vi "Read String Direct.vi"(8 "error in (no error)":errorcluster, 9 "Timeout (ms)":i32, 11 "CIFTag in":refnum<class "CIF_CIPC_Chn_String.lvclass">) -> (0 "error out":errorcluster, 1 "timed out?":bool, 2 "Data":string, 3 "CIFTag out":refnum<class "CIF_CIPC_Chn_String.lvclass">)   [LabVIEW 2021, in "CIF_CIPC_Chn_String.lvclass"]
uses:
  CIF_CIPC_Chn_String.lvclass
  D:/dev/Packages/CIF_Channels_Core/src/CIFChannels/CIFChannels.lvclass
  D:/dev/Packages/CIF_Channels_Core/src/CIPC_Channels/CIF_CIPC_Chan/CIF_CIPC_Chn.lvclass
  CIFChannels/CIFChannels.lvclass/CIFChannels.ctl
  ChannelCommon/typedef/Channel State.ctl
  ChannelCommon/typedef/Direction.ctl
  CIF_CIPC_Chn_String.lvclass/CIF_CIPC_Chn_String.ctl
  CIF_CIPC_Chan/CIF_CIPC_Chn.lvclass/CIF_CIPC_Chn.ctl
  561f6795-cf76-4d4d-b802-ea620fee8a5b.vi
  CIFChannels/Accessors/Read Channel State.vi
  CIFChannels/Accessors/Read Direction.vi
  CIFChannels/Accessors/Read Tag Forced.vi
  CIFChannels/Accessors/Write Channel State.vi
  CIFChannels/Accessors/Read Tag Disconnect Behavior.vi
  <vilib>/CIF Foundation/CIF CIPC/SubVIs/Wait For N Elements Available.vi
  <vilib>/CIF Foundation/CIF CIPC/SubVIs/Check Error.vi
  <vilib>/CIF Foundation/CIF CIPC/SubVIs/Get dll Path.vi
  <vilib>/CIF Foundation/CIF CIPC/SubVIs/Get Element Read Position.vi
  <vilib>/CIF Foundation/CIF CIPC/SubVIs/Set Element Read Position.vi
  CIF_CIPC_Chan/CIF_CIPC_Chn.lvclass
  <vilib>/CIF Foundation/CIF CIPC/SubVIs/Get Element Info Variant.vi
  <vilib>/CIF Foundation/CIF CIPC/SubVIs/Check Error Core.vi
  ChannelCommon/ChannelCommon.lvlib
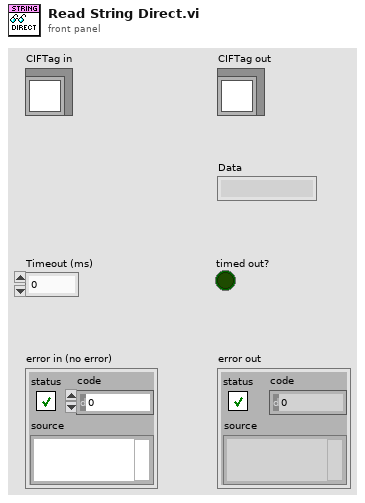
[diagram p1: front panel]
types:
  T1 = typedef "ChannelCommon.lvlib/Channel State.ctl" = enum8{"Creating", "Disconnected", "Connecting", "Connected", "Destroyed"}
  T2 = typedef "ChannelCommon.lvlib/Direction.ctl" = enum8{"Publisher", "Subscriber"}
  T3 = typedef "CIF_NI_CIPC.lvlib/Read Result Details.ctl" = cluster{"Array Size":i32, "Element Offset Last Read":u32, "Overwritten":bool, "Timeout":bool}
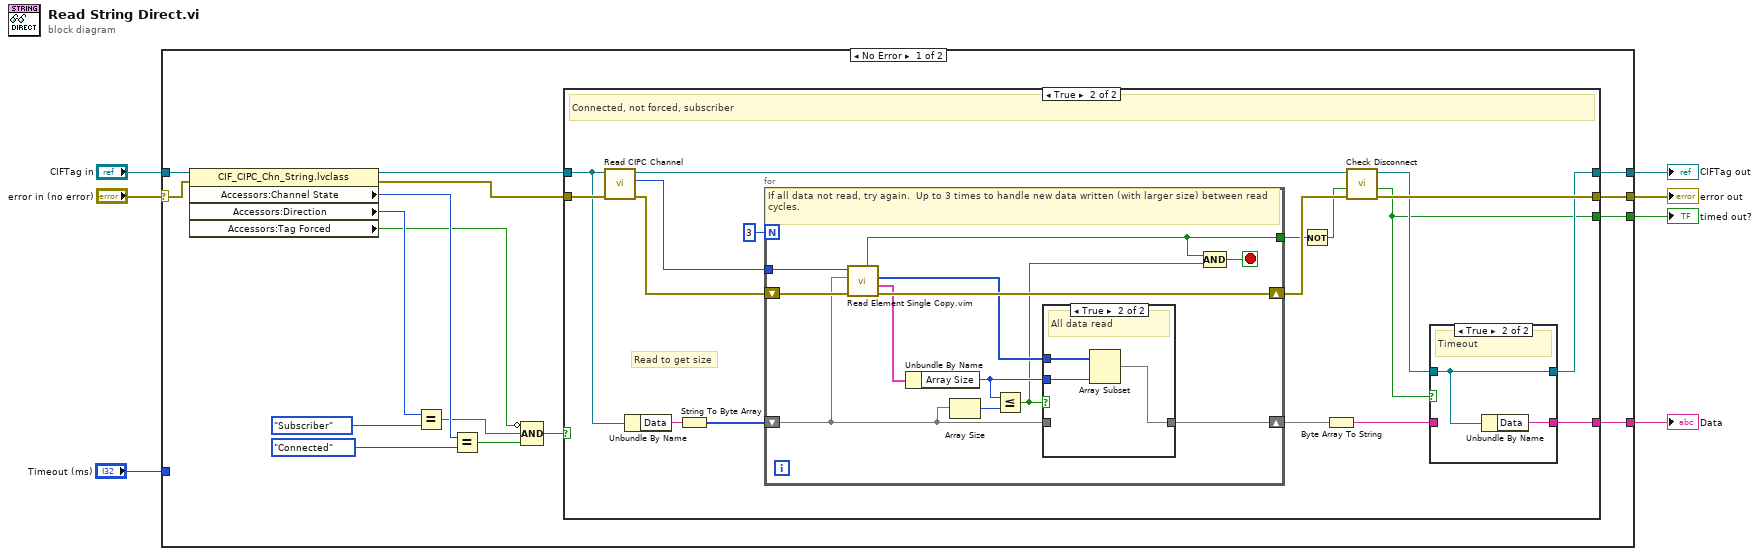
[diagram p0: block diagram]
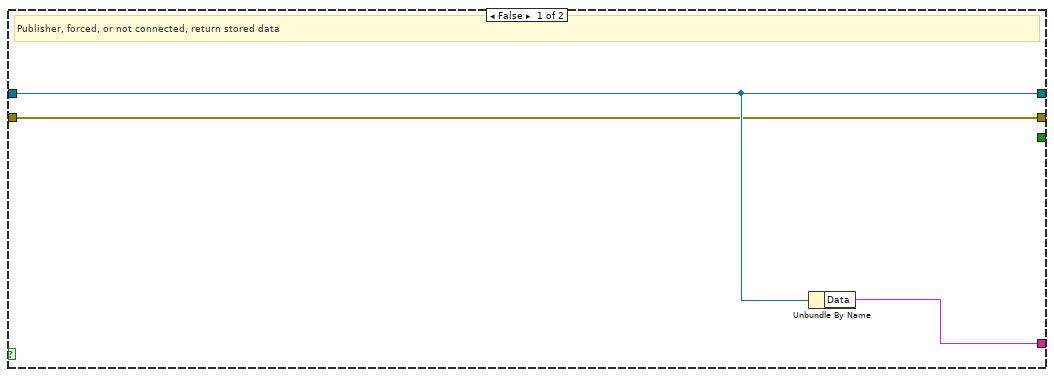
[diagram p2: hidden frame]
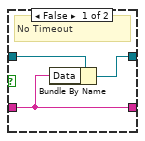
[diagram p3: hidden frame]
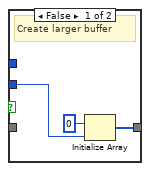
[diagram p4: hidden frame]
diagram:
  n1 = case shown="No Error" "error in (no error)" {
    selector: "error in (no error)" -> [w20 w69]
    tunnel: [w9 w69] -> w6
    tunnel: [w10 w68] -> w4
    tunnel: "CIFTag in" -> [w21 w68]
    tunnel: [w23 _] -> w3
    tunnel: [w22 _] -> w2
    tunnel: "Timeout (ms)" -> [_ _]
    frame No Error {
      n2 = property class="CIF_CIPC_Chn_String.lvclass"(reference=w21, error in=w20) -> (reference out=w19:refnum<class "CIF_CIPC_Chn_String.lvclass">, error out=w18:errorcluster, "Accessors:Channel State"=w15:T1, "Accessors:Direction"=w17:T2, "Accessors:Tag Forced"=w8:bool)
      n3 = Equal?(x=w17, y=Direction."Subscriber") -> (x = y?=w11:bool)
      n4 = Equal?(x=w15, y=Channel_State."Connected") -> (x = y?=w13:bool)
      n5 = Compound Arithmetic op=AND(invert w8, w11, w13) -> (w12:bool)
      n6 = case shown="True" w12 {
        tunnel: [_ w28] -> w23
        tunnel: [w26 w27] -> w22
        tunnel: w18 -> [w24 w44]
        tunnel: w19 -> [w25 w38]
        tunnel: [w25 w29] -> w10
        tunnel: [w24 w43] -> w9
        frame False {
          # "Publisher, forced, or not connected, return stored data"
          n7 = Unbundle By Name(w25) -> ("Data"=w26:string)
        }
        frame True {
          # "Read to get size"
          # "Connected, not forced, subscriber"
          n8 = call "Read CIPC Channel.vi"("error in (no error)"=w44, "CIFTag in"=w38) -> ("error out"=w41:errorcluster, "CIPC Channel"=w42:u64, "CIFTag out"=w31:refnum<class "CIF_CIPC_Chn_String.lvclass">)  [unwired: 7 in]
          n9 = Unbundle By Name(w38) -> ("Data"=w37:string)
          n10 = String To Byte Array(string=w37) -> (unsigned byte array=w36:u8[])
          n11 = for {
            N: 3 -> [_]
            tunnel: w42 -> [w61]
            tunnel: [w52] -> w39
            shift-right: [w59] -> w40
            shift-left: w41 -> [w60]
            shift-right: [w53] -> w35
            shift-left: w36 -> [w56]
            stop <- w51 stop-if-true
            # "If all data not read, try again.  Up to 3 times to handle new data written (with larger size) between read cycles."
            n12 = call "Read Element Single Copy.vim"("error in (no error)"=w60, "Data in"=w56, "CIPC Reference in"=w61) -> ("error out"=w59:errorcluster, "Read Result Details"=w55:T3, "Data out"=w54:u8[], "Success"=w52:bool)  [unwired: 4 in, 1 out]
            n13 = Unbundle By Name(w55) -> ("Array Size"=w57:i32)
            n14 = Array Size(array=w56) -> (size(s)=w58:i32)
            n15 = Less Or Equal?(x=w57, y=w58) -> (x <= y?=w50:bool)
            n16 = case shown="True" w50 {
              tunnel: w57 -> [w64 w66]
              tunnel: w56 -> [_ _]
              tunnel: [w62 w65] -> w53
              tunnel: w54 -> [_ w67]
              frame False {
                # "Create larger buffer"
                n17 = Initialize Array(u8 0 ("element"), w64) -> (w62:u8[])
              }
              frame True {
                # "All data read"
                n18 = Array Subset(array=w67, length=w66) -> (w65:u8[])  [unwired: 1 in]
              }
            }
            n19 = Compound Arithmetic op=AND(w52, w50) -> (w51:bool)
          }
          n20 = Not(x=w39) -> (.not. x?=w32:bool)
          n21 = Byte Array To String(unsigned byte array=w35) -> (string=w34:string)
          n22 = call "Check Disconnect.vi"("error in (no error)"=w40, "timeout in"=w32, "CIFTag in"=w31) -> ("error out"=w43:errorcluster, "timeout out"=w28:bool, "CIFTag out"=w30:refnum<class "CIF_CIPC_Chn_String.lvclass">)  [unwired: 5 in, 1 out]
          n23 = case shown="True" w28 {
            tunnel: w34 -> [w45 _]
            tunnel: w30 -> [w47 w49]
            tunnel: [w46 w49] -> w29
            tunnel: [w45 w48] -> w27
            frame False {
              # "No Timeout"
              n24 = Bundle By Name(cluster=w47, "Data"=w45) -> (w46:refnum<class "CIF_CIPC_Chn_String.lvclass">)
            }
            frame True {
              # "Timeout"
              n25 = Unbundle By Name(w49) -> ("Data"=w48:string)
            }
          }
        }
      }
    }
    frame Error {
    }
  }
  "error out" <- w6
  "CIFTag out" <- w4
  "timed out?" <- w3
  "Data" <- w2
